vi "fittingParams.vi"(5 "read/write":T1, 7 "error in (no error)":errorcluster, 8 "setpoints":T2={"target clarified turbidity (NTU)"=0.3, "flocculator volume (L)"=0.0, "clarifier volume (L)"=0.0, "dose updates per HRT"=1} {"target clarified turbidity (NTU)" min=0.1 max=5.0 step=0.01; "dose updates per HRT" min=1 max=1000 step=1}) -> (0 "error out":errorcluster, 1 "Ccoag-DOM":dbl, 2 "Ku*":dbl, 3 "Fitting Params":cluster{dbl[], "Best Linear Fit":dbl[]}[](graph))   [LabVIEW 2014]
uses:
  ProCoDA/DAQ configuration/Sensor buffer command.ctl
  <vilib>/Analysis/NI_AALPro.lvlib
  setpoints.ctl
  calcDoseorGetGraph.ctl
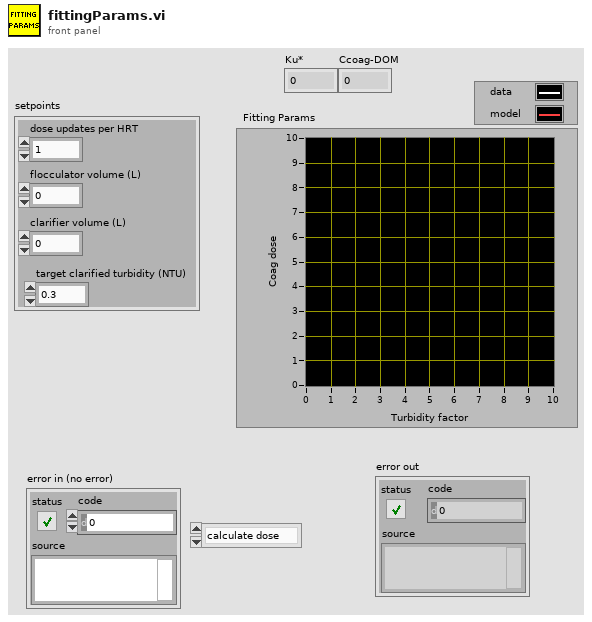
[diagram p1: front panel]
types:
  T1 = typedef "calcDoseorGetGraph.ctl" = enum16{"calculate dose", "read graph"}
  T2 = typedef "setpoints.ctl" = cluster{"target clarified turbidity (NTU)":dbl, "flocculator volume (L)":dbl, "clarifier volume (L)":dbl, "dose updates per HRT":u32}
  T3 = typedef "Sensor buffer command.ctl" = enum16{"set buffer size", "write", "refill buffer", "read recent", "read all", "clear"}
  T4 = typedef "data cluster.ctl" = cluster{"Clarified turbidity (NTU)":dbl, "Raw turbidity (NTU)":dbl, "flow rate (L/s)":dbl, "time":timestamp}
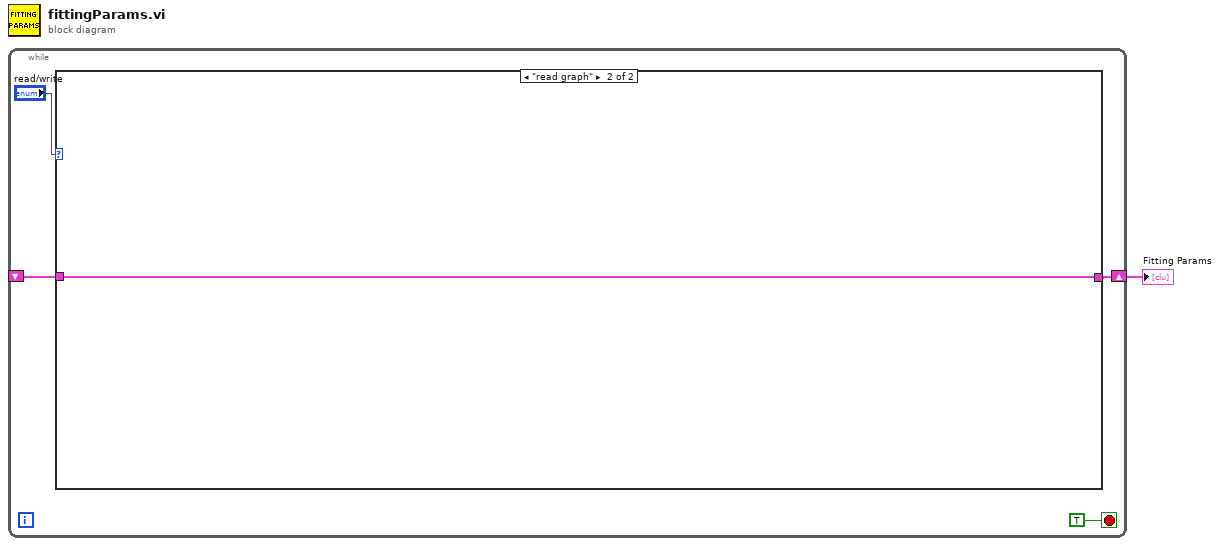
[diagram p0: block diagram]
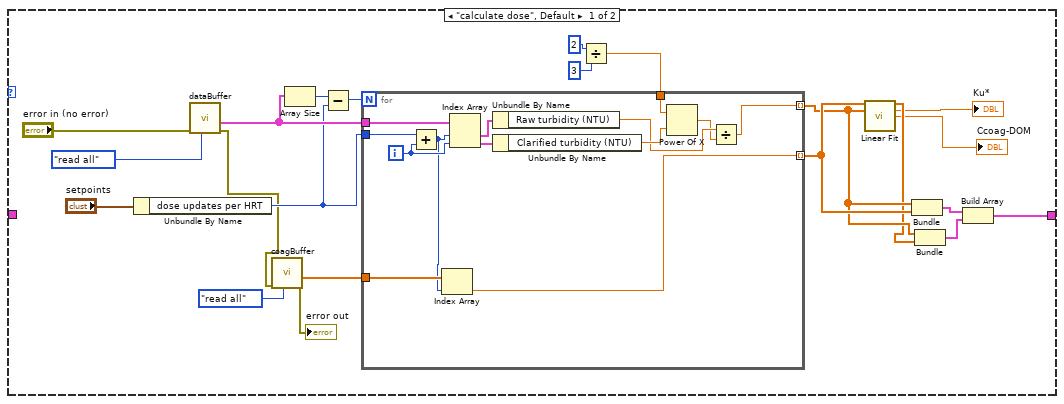
[diagram p2: hidden frame]
diagram:
  n1 = while {
    shift-right: [w5] -> w1
    shift-left: _ -> [w4]
    stop <- TRUE stop-if-true
    n2 = case shown="\"read graph\"" "read/write" {
      tunnel: [w11 w41] -> w5
      tunnel: w4 -> [_ w41]
      frame "calculate dose", Default {
        n3 = Unbundle By Name("setpoints") -> ("dose updates per HRT"=w22:u32)
        n4 = call "dataBuffer.vi"("command"=Sensor_buffer_command."read all", "error in (no error)"="error in (no error)") -> ("error out"=w7:errorcluster, "all data out"=w25:T4[])  [unwired: 7 in, 1 out]
        n5 = call "coagBuffer.vi"("command"=Sensor_buffer_command."read all", "error in (no error)"=w7) -> ("error out"=→"error out":errorcluster, "all coag out"=w17:dbl[])  [unwired: 7 in, 1 out]
        n6 = Array Size(array=w25) -> (size(s)=w23:i32)
        n7 = Subtract(x=w23, y=w22) -> (x-y=w24:u32)
        n8 = Divide(x=2, y=3) -> (x/y=w19:dbl)
        n9 = for {
          N: w24 -> [_]
          tunnel: w25 -> [w40]
          tunnel: w22 -> [w39]
          tunnel: w19 -> [w35]
          tunnel: w17 -> [w31]
          tunnel: [w29] -> w15 mode=indexing
          tunnel: [w28] -> w16 mode=indexing
          i -> [w38]
          n10 = Add(x=w39, y=w38) -> (x+y=w30:u32)
          n11 = Index Array(array=w31, index=w30) -> (element=w28:dbl)
          n12 = Index Array(array=w40, index #1=w30, index #2=w38) -> (element #1=w37:T4, element #2=w36:T4)
          n13 = Unbundle By Name(w37) -> ("Raw turbidity (NTU)"=w33:dbl)
          n14 = Unbundle By Name(w36) -> ("Clarified turbidity (NTU)"=w34:dbl)
          n15 = Power Of X(1:w34, 2:w35) -> (0:w32:dbl)
          n16 = Divide(x=w33, y=w32) -> (x/y=w29:dbl)
        }
        n17 = call <vilib>:"Linear Fit.vi"("Y"=w16, "X"=w15) -> ("Best Linear Fit"=w14:dbl[], "slope"=→"Ku*":dbl, "intercept"=→"Ccoag-DOM":dbl)  [unwired: 9 in, 2 out]
        n18 = Bundle(w15, w16) -> (w13:cluster{dbl[], dbl[]})  [unwired: 1 in]
        n19 = Bundle(w15, "Best Linear Fit"=w14) -> (w12:cluster{dbl[], "Best Linear Fit":dbl[]})  [unwired: 1 in]
        n20 = Build Array(w13, w12) -> (w11:cluster{dbl[], "Best Linear Fit":dbl[]}[])
      }
      frame "read graph" {
      }
    }
  }
  "Fitting Params" <- w1
